vi "output-save-ibw-wavelist.vi"(0 "BG Wave Name":string, 1 "Abort?":bool=TRUE, 3 "PL Wave Name":string, 4 "Loop Indicator":i32, 5 "select background":enum16{"skip", "single", "multiple"}(ring)) -> (2 "Complete Wave List String":string)   [LabVIEW 2015]
panel:
  out "Combined Wave Names":string
  out "Loop/Column Numbers":string
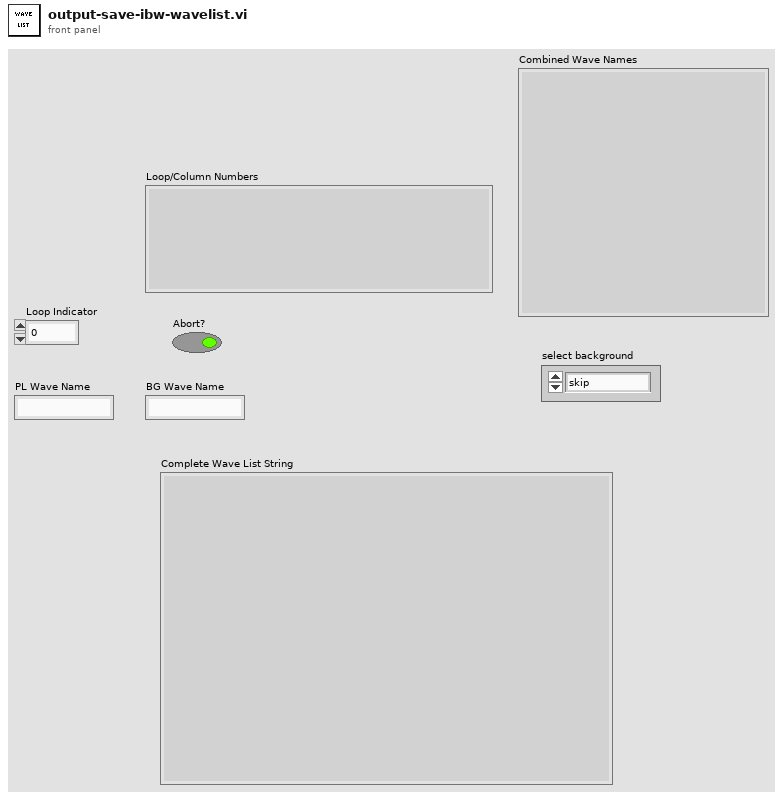
[diagram p1: front panel]
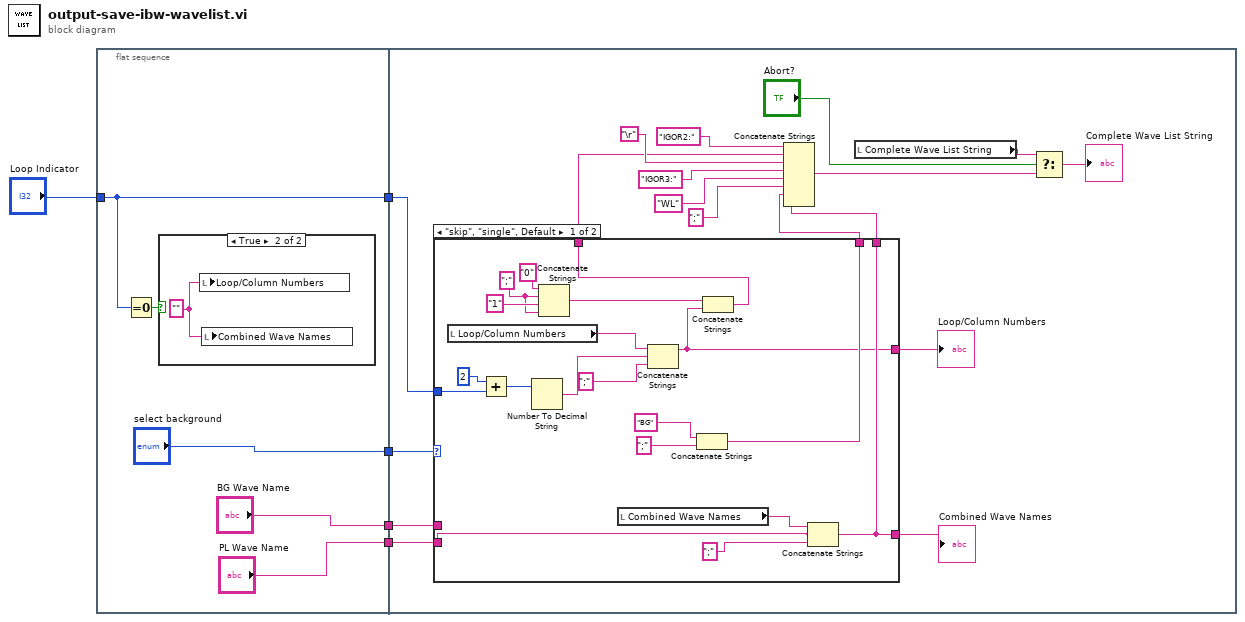
[diagram p0: block diagram]
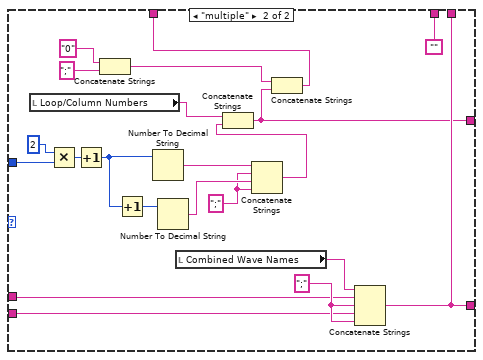
[diagram p3: hidden frame]
diagram:
  n1 = flat-sequence {
    tunnel: "Loop Indicator" -> [w9]
    tunnel: [w9] -> w5
    tunnel: ["PL Wave Name"] -> w4
    tunnel: ["BG Wave Name"] -> w3
    tunnel: ["select background"] -> w2
    tunnel: w5 -> [w14]
    tunnel: w4 -> [w17]
    tunnel: w3 -> [w16]
    tunnel: w2 -> [w15]
    frame #0 {
      n2 = Equal To 0?(x=w9) -> (x = 0?=w10:bool)
      n3 = case shown="True" w10 {
        frame False {
        }
        frame True {
          w11 = "" ("concatenated string")
          n4 = local write "Loop/Column Numbers"(w11) -> ()
          n5 = local write "Combined Wave Names"(w11) -> ()
        }
      }
    }
    frame #1 {
      n6 = case shown="\"skip\", \"single\", Default" w15 {
        tunnel: [w47 w67] -> w24
        tunnel: [w47 w67] -> w23
        tunnel: [w44 ""] -> w18
        tunnel: w17 -> [w33 w64]
        tunnel: w16 -> [_ w65]
        tunnel: w14 -> [w39 w59]
        tunnel: [w36 w52] -> w13
        tunnel: [w34 w50] -> w12
        frame "skip", "single", Default {
          w41 = ";"
          n7 = local read "Loop/Column Numbers"() -> (w40:string)
          n8 = Add(x=2, y=w39) -> (x+y=w38:i32)
          n9 = Number To Decimal String(number=w38) -> (decimal integer string=w31:string)  [unwired: 1 in]
          n10 = Concatenate Strings("0", w41, "1", w41) -> (w35:string)
          n11 = local read "Combined Wave Names"() -> (w48:string)
          n12 = Concatenate Strings(w40, w31, ";") -> (w36:string)
          n13 = Concatenate Strings("BG", ";") -> (w44:string)
          n14 = Concatenate Strings(w35, w36) -> (w34:string)
          n15 = Concatenate Strings(w48, w33, ";") -> (w47:string)
        }
        frame "multiple" {
          w53 = ";"
          w68 = ";"
          n16 = local read "Loop/Column Numbers"() -> (w56:string)
          n17 = Multiply(x=2, y=w59) -> (x*y=w60:i32)
          n18 = Increment(x=w60) -> (x+1=w58:i32)
          n19 = Concatenate Strings("0", ";") -> (w51:string)
          n20 = Increment(x=w58) -> (x+1=w57:i32)
          n21 = Number To Decimal String(number=w58) -> (decimal integer string=w55:string)  [unwired: 1 in]
          n22 = Number To Decimal String(number=w57) -> (decimal integer string=w54:string)  [unwired: 1 in]
          n23 = local read "Combined Wave Names"() -> (w66:string)
          n24 = Concatenate Strings(w55, w53, w54, w53) -> (w49:string)
          n25 = Concatenate Strings(w56, w49) -> (w52:string)
          n26 = Concatenate Strings(w51, w52) -> (w50:string)
          n27 = Concatenate Strings(w66, w65, w68, w64, w68) -> (w67:string)
        }
      }
      "Combined Wave Names" <- w24
      "Loop/Column Numbers" <- w13
      n28 = Concatenate Strings("IGOR2:", w12, "\r", "IGOR3:", "WL", ";", w18, w23) -> (w22:string)
      n29 = local read "Complete Wave List String"() -> (w20:string)
      n30 = Select(t=w20, s="Abort?", f=w22) -> (s? t:f=→"Complete Wave List String":string)
    }
  }
